vi "cno_adjust OB for IC.vi"(5 "cno data":T1, 7 "P":dbl[](array[numeric]), 8 "error in (no error)":errorcluster, 11 "OB":dbl[](array[numeric])) -> (0 "error out":errorcluster, 3 "OB":dbl[](array[numeric]))   [LabVIEW 2014, in "NI_Gmath.lvlib"]
uses:
  NI_Gmath.lvlib
  cno_data.ctl
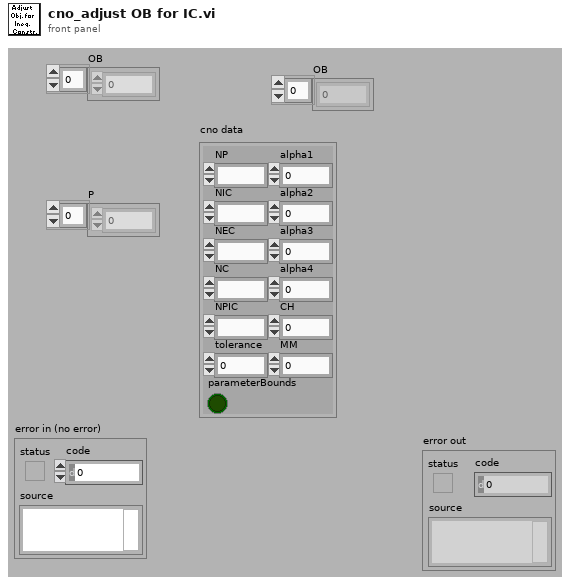
[diagram p1: front panel]
types:
  T1 = typedef "NI_Gmath.lvlib/cno_data.ctl" = cluster{"NP":i32, "NIC":i32, "NEC":i32, "NC":i32, "NPIC":i32, "parameterBounds":bool, "alpha1":dbl, "alpha2":dbl, "alpha3":dbl, "alpha4":dbl, "CH":i32, "MM":i32, "tolerance":dbl}
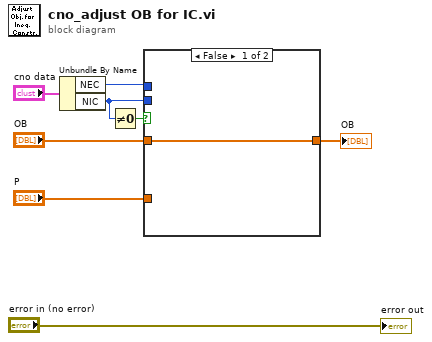
[diagram p0: block diagram]
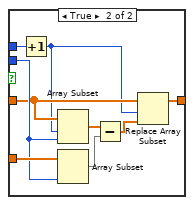
[diagram p2: hidden frame]
diagram:
  n1 = Unbundle By Name("cno data") -> ("NEC"=w3:i32, "NIC"=w2:i32)
  n2 = Not Equal To 0?(x=w2) -> (x != 0?=w5:bool)
  n3 = case shown="False" w5 {
    tunnel: "P" -> [_ w17]
    tunnel: "OB" -> [w9 w13]
    tunnel: w3 -> [_ w18]
    tunnel: w2 -> [_ w16]
    tunnel: [w9 w10] -> w8
    frame False {
    }
    frame True {
      n4 = Increment(x=w18) -> (x+1=w12:i32)
      n5 = Array Subset(array=w13, index=w12, length=w16) -> (w15:dbl[])
      n6 = Array Subset(array=w17, length=w16) -> (w14:dbl[])  [unwired: 1 in]
      n7 = Subtract(x=w15, y=w14) -> (x-y=w11:dbl[])
      n8 = Replace Array Subset(array=w13, new element=w11, index=w12) -> (w10:dbl[])
    }
  }
  "OB" <- w8
  "error out" <- "error in (no error)"
